vi "Find Important Module VIs paths.vi"(11 "Library in":refnum<vi>) -> (3 "Public API VIs Paths":path[](array[path]))   [LabVIEW 2019, in "Panther Dashboard.lvlib"]
uses:
  Panther Dashboard.lvlib
  Public VIs names--enum.ctl
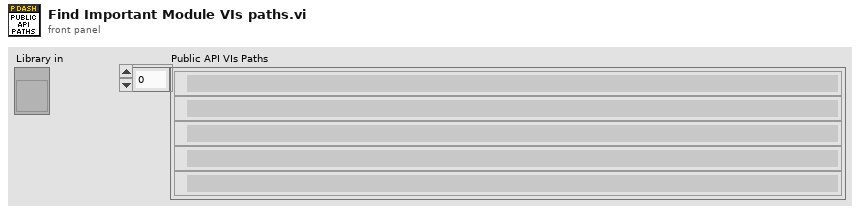
[diagram p1: front panel]
types:
  T1 = typedef "Panther Dashboard.lvlib/Public VIs names--enum.ctl" = enum16{"Start Module.vi", "Synchronize Module Events.vi", "Obtain Broadcast Events for Registration.vi", "Null Broadcast Events--constant.vi", "Stop Module.vi"}
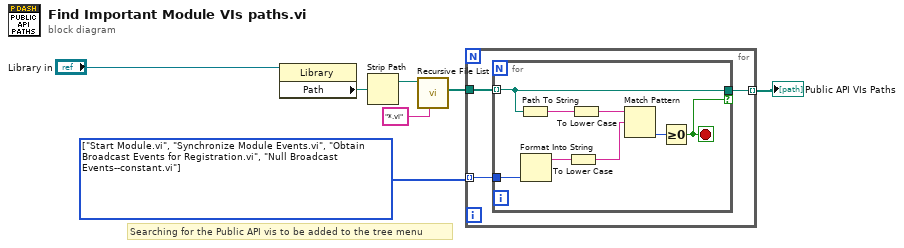
[diagram p0: block diagram]
diagram:
  w6 = T1[] [enum."Start Module.vi", enum."Synchronize Module Events.vi", enum."Obtain Broadcast Events for Registration.vi", enum."Null Broadcast Events--constant.vi"] items=["Start Module.vi", "Synchronize Module Events.vi", "Obtain Broadcast Events for Registration.vi", "Null Broadcast Events--constant.vi", "Stop Module.vi"]
  # "Searching for the Public API vis to be added to the tree menu"
  n1 = property class="Library"(reference="Library in") -> ("Path"=w3:path)  [unwired: 1 in, 2 out]
  n2 = Strip Path(path=w3) -> (stripped path=w2:path)  [unwired: 1 out]
  n3 = call <vilib>:"Recursive File List.vi"("pattern"="*.vi", "Folder Path"=w2) -> ("All Files in Dir"=w5:path[])  [unwired: 5 in, 4 out]
  n4 = for {
    tunnel: w6 -> [w10] mode=indexing
    tunnel: w5 -> [w9]
    tunnel: [w8] -> w4 mode=indexing
    n5 = for {
      tunnel: w10 -> [w18]
      tunnel: w9 -> [w14] mode=indexing
      tunnel: [w14] -> w8 if=w13
      stop <- w13 stop-if-true
      n6 = Path To String(path=w14) -> (string=w16:string)
      n7 = Format Into String(w18) -> (resulting string=w17:string)  [unwired: 3 in, 1 out]
      n8 = To Lower Case(string=w17) -> (all lower case string=w11:string)
      n9 = To Lower Case(string=w16) -> (all lower case string=w12:string)
      n10 = Match Pattern(string=w12, regular expression=w11) -> (offset past match=w15:i32)  [unwired: 1 in, 3 out]
      n11 = Greater Or Equal To 0?(x=w15) -> (x >= 0?=w13:bool)
    }
  }
  "Public API VIs Paths" <- w4
